vi "LimitTemplatesToFilter.vi"(10 "Filter":string="Desktop:Templates", 11 "Templates In":refnum<class "MetaDataObj.lvclass">[](array[class])) -> (3 "Templates Out":refnum<class "MetaDataObj.lvclass">[](array[class]))   [LabVIEW 2016, in "NI_NPW_Filters.lvlib"]
uses:
  <resource>/dialog/NewProjectWizard/Filters/NI_NPW_Filters.lvlib
  <resource>/dialog/NewProjectWizard/MetaDataObj/MetaDataObj.lvclass
  <resource>/dialog/NewProjectWizard/MetaDataObj/Accessors/Read Filters.vi
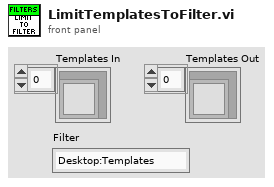
[diagram p1: front panel]
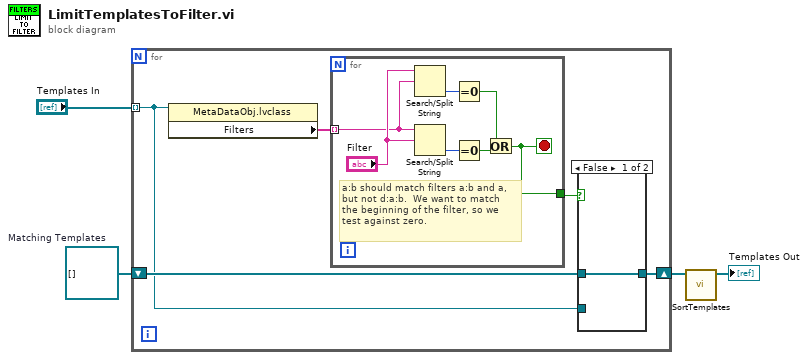
[diagram p0: block diagram]
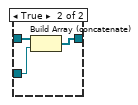
[diagram p2: hidden frame]
diagram:
  w3 = refnum<class "MetaDataObj.lvclass">[] []  # Matching Templates
  n1 = for {
    tunnel: "Templates In" -> [w5] mode=indexing
    shift-right: [w6] -> w2
    shift-left: w3 -> [w7]
    n2 = property class="MetaDataObj.lvclass"(reference=w5) -> ("Filters"=w9:string[])  [unwired: 1 in, 2 out]
    n3 = for {
      tunnel: w9 -> [w17] mode=indexing
      tunnel: [w14] -> w8
      stop <- w14 stop-if-true
      # "a:b should match filters a:b and a,\nbut not d:a:b.  We want to match\nthe beginning of the filter, so we\ntest against zero."
      n4 = Search/Split String(string="Filter", search string/char (-)=w17) -> (offset of match=w19:i32)  [unwired: 1 in, 2 out]
      n5 = Search/Split String(string=w17, search string/char (-)="Filter") -> (offset of match=w20:i32)  [unwired: 1 in, 2 out]
      n6 = Equal To 0?(x=w19) -> (x = 0?=w15:bool)
      n7 = Equal To 0?(x=w20) -> (x = 0?=w16:bool)
      n8 = Or(x=w15, y=w16) -> (x .or. y?=w14:bool)
    }
    n9 = case shown="False" w8 {
      tunnel: w7 -> [w10 w13]
      tunnel: [w10 w11] -> w6
      tunnel: w5 -> [_ w12]
      frame False {
      }
      frame True {
        n10 = Build Array (concatenate)(w13, w12) -> (w11:refnum<class "MetaDataObj.lvclass">[])
      }
    }
  }
  n11 = call <resource>:"SortTemplates.vi"("Unsorted Templates"=w2) -> ("Sorted Templates"=→"Templates Out":refnum<class "MetaDataObj.lvclass">[])  [unwired: 10 in]
